vi "grab_qrcode.vi"() -> ()   [LabVIEW 2018]
uses:
  0460686a-1f5f-4a7d-b7f5-93a42d0cd41c.vi
panel:
  out "filename":string
  in  "stop":bool
  out "Input QR Code":picture
  out "Output QR Code":picture
  out "return value":cluster{"found":i32, "decode data":string}
  in  "Output image filename":string="decode.png"
  in  "QR Code Image Path":string="qrcode_src"
  # "Free QR code generator website"
  # "https://www.the-qrcode-generator.com/"
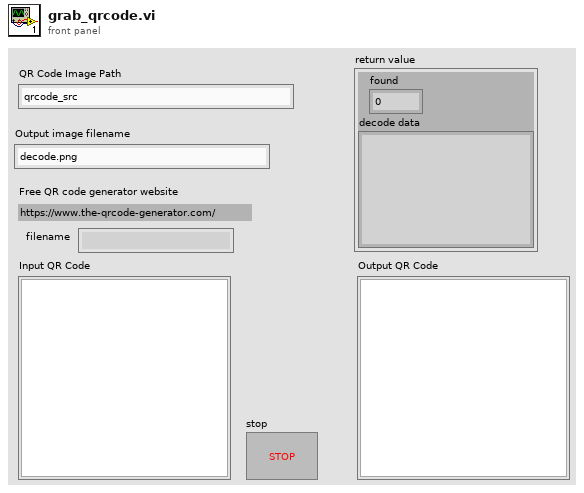
[diagram p1: front panel]
types:
  T1 = typedef "imagedata.ctl" = cluster{"image type":i32, "image depth":i32, "image":u8[], "mask":u8[], "colors":u32[], "Rectangle":cluster{"left":i16, "top":i16, "right":i16, "bottom":i16}}
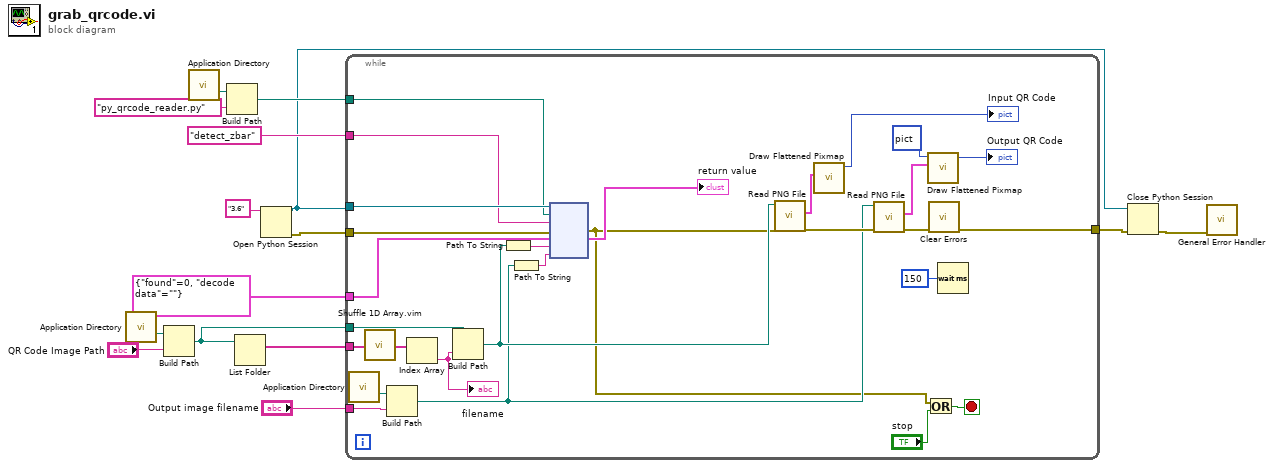
[diagram p0: block diagram]
diagram:
  n1 = call <vilib>:"Application Directory.vi"() -> ("Application Directory"=w6:path)
  n2 = Build Path(base path=w6, name or relative path="QR Code Image Path") -> (appended path=w4:path)
  n3 = call <vilib>:"Application Directory.vi"() -> ("Application Directory"=w12:path)
  n4 = Build Path(base path=w12, name or relative path="py_qrcode_reader.py" ("module filename")) -> (appended path=w10:path)
  n5 = List Folder(path=w4) -> (filenames=w9:string[])  [unwired: 3 in, 3 out]
  n6 = Open Python Session(python version="3.6" ("Python version")) -> (session out=w2:refnum<k35>, error out=w3:errorcluster)  [unwired: 2 in]
  n7 = while {
    tunnel: w2 -> [w43]
    tunnel: w3 -> [w42]
    tunnel: "detect_zbar" ("function name") -> [w41]
    tunnel: cluster{"found":i32, "decode data":string} {"found"=0, "decode data"=""} -> [w40]
    tunnel: "Output image filename" -> [w20]
    tunnel: w10 -> [w35]
    tunnel: w4 -> [w26]
    tunnel: w9 -> [w31]
    tunnel: [w22] -> w8
    stop <- w28 stop-if-true
    n8 = call <vilib>:"Application Directory.vi"() -> ("Application Directory"=w38:path)
    n9 = call "Shuffle 1D Array.vim"("array"=w31) -> ("shuffled array"=w30:string[])  [unwired: 4 in]
    n10 = Build Path(base path=w38, name or relative path=w20) -> (appended path=w18:path)
    n11 = Index Array(array=w30) -> (element=w23:string)  [unwired: 1 in]
    "filename" <- w23
    n12 = Build Path(base path=w26, name or relative path=w23) -> (appended path=w25:path)
    n13 = Path To String(path=w25) -> (string=w24:string)
    n14 = Path To String(path=w18) -> (string=w19:string)
    n15 = node(w43, w35, w41, w42, w40, w24, w19) -> (w17:errorcluster, →"return value":cluster{"found":i32, "decode data":string})  [unwired: 2 in, 3 out]
    n16 = call <vilib>:"Read PNG File.vi"("error in (no error)"=w17, "path to PNG file"=w25) -> ("error out"=w34:errorcluster, "image data"=w33:T1)  [unwired: 7 in, 1 out]
    n17 = call <vilib>:"Draw Flattened Pixmap.vi"("image data"=w33) -> ("new picture"=→"Input QR Code":picture)  [unwired: 8 in]
    n18 = call <vilib>:"Read PNG File.vi"("error in (no error)"=w34, "path to PNG file"=w18) -> ("error out"=w27:errorcluster, "image data"=w37:T1)  [unwired: 7 in, 1 out]
    n19 = Or(x=w17, y="stop") -> (x .or. y?=w28:bool)
    n20 = call <vilib>:"Draw Flattened Pixmap.vi"("image data"=w37, "picture"=picture data[5B]) -> ("new picture"=→"Output QR Code":picture)  [unwired: 7 in]
    n21 = call <vilib>:"Clear Errors.vi"("error in (no error)"=w27) -> ("error out"=w22:errorcluster)  [unwired: 5 in, 1 out]
    n22 = Wait (ms)(milliseconds to wait=u32 150) -> ()  [unwired: 1 out]
  }
  n23 = Close Python Session(session in=w2, error in=w8) -> (11:w7:errorcluster)
  n24 = call <vilib>:"General Error Handler.vi"("error in (no error)"=w7) -> ()  [unwired: 10 in, 5 out]
